vi "REV2mDistanceSensor FGV.vi"(6 "Port":T1=enum."MXP", 7 "Operation":enum16{"set", "get"}(ring), 8 "error in":errorcluster, 9 "Range":dbl format="%#_13g", 10 "Sensor Ready?":bool, 11 "REV2mDistanceSensorsArray":T2) -> (0 "error out":errorcluster, 1 "Range":dbl, 2 "Range Valid":bool, 3 "REV2mDistanceSensorsArray Out":T2)   [LabVIEW 2019, in "DistanceSensorDriver.lvlib"]
uses:
  DistanceSensorDriver.lvlib
  Typedef/Rev2mDistanceSensorsArray.ctl
  Typedef/REV2mDistanceSensorDevRef.ctl
  Typedef/Ports.ctl
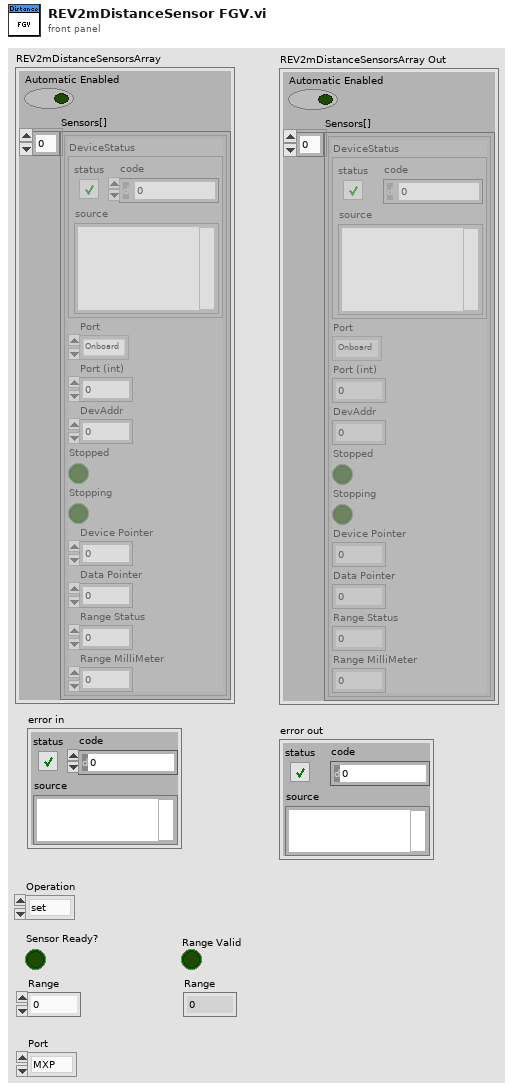
[diagram p1: front panel]
types:
  T1 = typedef "DistanceSensorDriver.lvlib/Ports.ctl" = enum32{"Onboard", "MXP"}
  T2 = typedef "DistanceSensorDriver.lvlib/Rev2mDistanceSensorsArray.ctl" = cluster{"Automatic Enabled":bool, "Sensors[]":T3[]}
  T3 = typedef "DistanceSensorDriver.lvlib/REV2mDistanceSensorDevRef.ctl" = cluster{"DeviceStatus":errorcluster, "Port":T1, "Port (int)":i32, "DevAddr":i32, "Stopped":bool, "Stopping":bool, "Device Pointer":u64, "Data Pointer":u64, "Range Status":u8, "Range MilliMeter":u16}
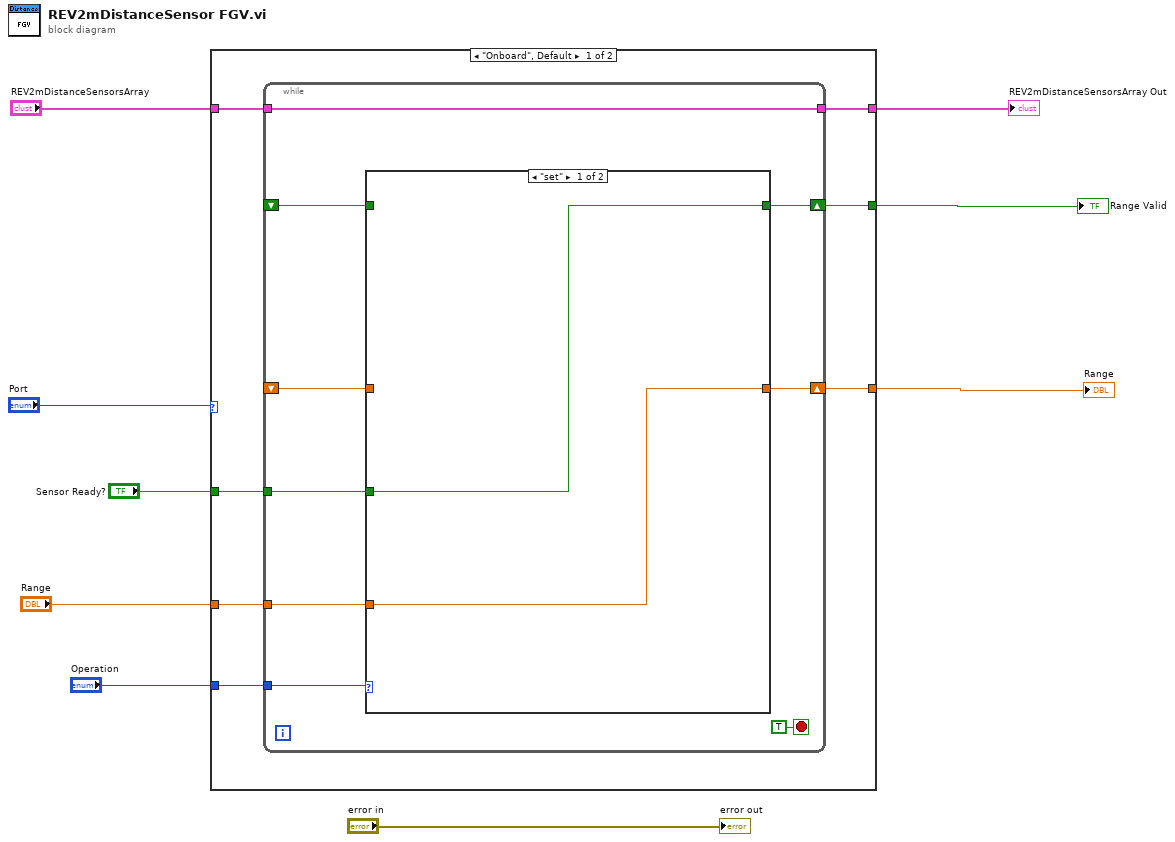
[diagram p0: block diagram]
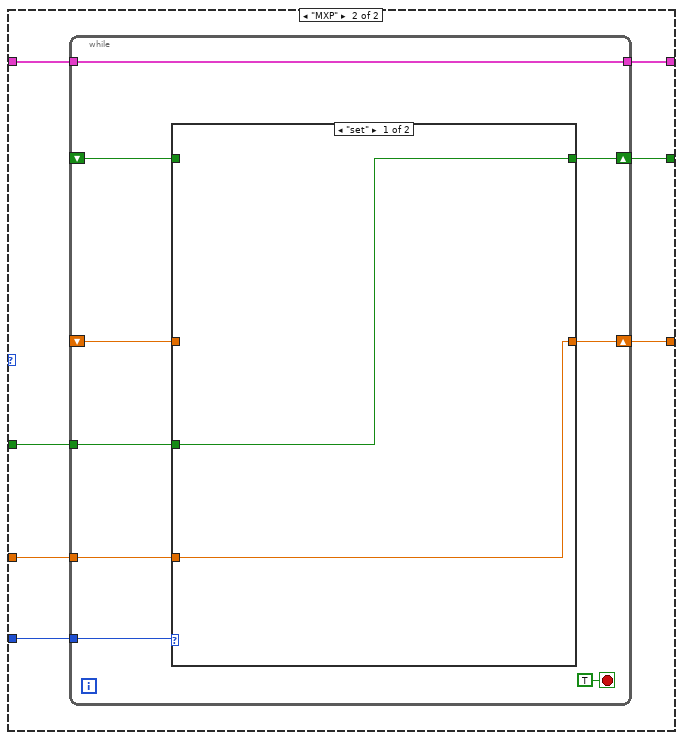
[diagram p3: hidden frame]
diagram:
  n1 = case shown="\"Onboard\", Default" "Port" {
    tunnel: [w16 w36] -> w9
    tunnel: [w15 w35] -> w7
    tunnel: "Operation" -> [w14 w34]
    tunnel: "REV2mDistanceSensorsArray" -> [w13 w33]
    tunnel: [w12 w32] -> w3
    tunnel: "Sensor Ready?" -> [w11 w31]
    tunnel: "Range" -> [w10 w30]
    frame "Onboard", Default {
      n2 = while {
        shift-right: [w23] -> w16
        shift-left: _ -> [w24]
        shift-right: [w22] -> w15
        shift-left: _ -> [w21]
        tunnel: w14 -> [w20]
        tunnel: w13 -> [w19]
        tunnel: [w19] -> w12
        tunnel: w11 -> [w18]
        tunnel: w10 -> [w17]
        stop <- TRUE stop-if-true
        n3 = case shown="\"set\"" w20 {
          tunnel: [w27 w29] -> w23
          tunnel: w24 -> [_ w29]
          tunnel: [w26 w28] -> w22
          tunnel: w21 -> [_ w28]
          tunnel: w18 -> [w27 _]
          tunnel: w17 -> [w26 _]
          frame "set" {
          }
          frame "get", Default {
          }
        }
      }
    }
    frame "MXP" {
      n4 = while {
        shift-right: [w43] -> w36
        shift-left: _ -> [w44]
        shift-right: [w42] -> w35
        shift-left: _ -> [w41]
        tunnel: w34 -> [w40]
        tunnel: w33 -> [w39]
        tunnel: [w39] -> w32
        tunnel: w31 -> [w38]
        tunnel: w30 -> [w37]
        stop <- TRUE stop-if-true
        n5 = case shown="\"set\"" w40 {
          tunnel: [w47 w49] -> w43
          tunnel: w44 -> [_ w49]
          tunnel: [w46 w48] -> w42
          tunnel: w41 -> [_ w48]
          tunnel: w38 -> [w47 _]
          tunnel: w37 -> [w46 _]
          frame "set" {
          }
          frame "get", Default {
          }
        }
      }
    }
  }
  "Range Valid" <- w9
  "Range" <- w7
  "REV2mDistanceSensorsArray Out" <- w3
  "error out" <- "error in"
